vi "se_mot_calc.vi"(6 "targetValid":bool=TRUE, 7 "resetOrigin":bool, 8 "inputValid":bool, 9 "interpOutput":fxp<+/-,19,2>, 10 "origin":T2, 11 "se.mot.p.target":cluster{"x":fxp<+/-,16,1>, "y":fxp<+/-,16,1>}) -> (0 "outputValid":bool, 2 "outputNorm":T1, 3 "outputInt":cluster{"x":i16, "y":i16})   [LabVIEW 2016]
uses:
  <vilib>/rvi/FXPMathLib/FxpSub/XNode/nifxpmath_Sub.xnode
  <vilib>/rvi/FXPMathLib/FxpMul/XNode/nifxpmath_Multiplier.xnode
  <vilib>/rvi/FXPMathLib/FxpAdd/XNode/nifxpmath_Add.xnode
  <vilib>/rvi/FXPMathLib/FxpInterpret/XNode/nifxpmath_Interpret.xnode
  <vilib>/rvi/FXPMathLib/sim/FxpSim.dll
types:
  T1 = cluster{"x+y":fxp<+/-,18,2>, "x+y":fxp<+/-,18,2>}
  T2 = cluster{"xOut":fxp<+/-,18,2>, "yOut":fxp<+/-,18,2>}
  T3 = cluster{"x-y":fxp<+/-,18,2>, "x-y":fxp<+/-,18,2>}
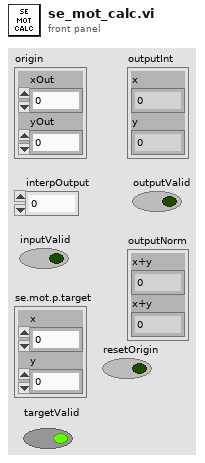
[diagram p1: front panel]
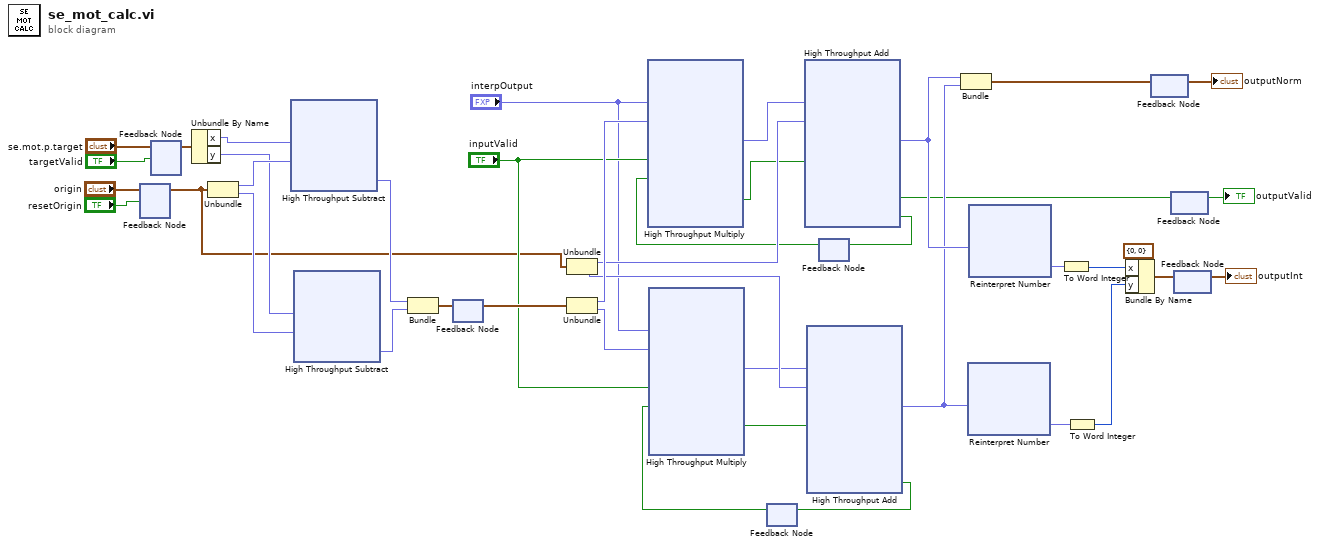
[diagram p0: block diagram]
diagram:
  n1 = feedback-in #1("origin", "resetOrigin") -> ()
  n2 = feedback #1() -> (w2:T2)  [unwired: 1 in]
  n3 = feedback-in #2("se.mot.p.target", "targetValid") -> ()
  n4 = feedback #2() -> (w6:cluster{"x":fxp<+/-,16,1>, "y":fxp<+/-,16,1>})  [unwired: 1 in]
  n5 = Unbundle By Name(w6) -> ("x"=w21:fxp<+/-,16,1>, "y"=w20:fxp<+/-,16,1>)
  n6 = Unbundle(w2) -> ("xOut"=w29:fxp<+/-,18,2>, "yOut"=w28:fxp<+/-,18,2>)
  n7 = xnode "High Throughput Subtract"("x"=w21, "y"=w29) -> ("x-y"=w35:fxp<+/-,18,2>)
  n8 = xnode "High Throughput Subtract"("x"=w20, "y"=w28) -> ("x-y"=w36:fxp<+/-,18,2>)
  n9 = Bundle("x-y"=w35, "x-y"=w36) -> (w37:T3)  [unwired: 1 in]
  n10 = feedback #3() -> (w38:T3)  [unwired: 1 in]
  n11 = feedback-in #3(w37) -> ()
  n12 = Unbundle(w2) -> ("xOut"=w34:fxp<+/-,18,2>, "yOut"=w33:fxp<+/-,18,2>)
  n13 = Unbundle(w38) -> ("x-y"=w41:fxp<+/-,18,2>, "x-y"=w40:fxp<+/-,18,2>)
  n14 = feedback #4() -> (w18:bool)  [unwired: 1 in]
  n15 = xnode ("High Throughput Multiply")("x"="interpOutput", "y"=w40, "input valid"="inputValid", "ready for output (T)"=w18) -> ("x*y"=w13:fxp<+/-,18,2>, "output valid"=w12:bool)  [unwired: 1 out]
  n16 = xnode ("High Throughput Add")("x"=w13, "y"=w33, "input valid"=w12) -> ("x+y"=w25:fxp<+/-,18,2>, "ready for input"=w19:bool)  [unwired: 1 in, 1 out]
  n17 = feedback-in #4(w19) -> ()
  n18 = feedback #5() -> (w16:bool)  [unwired: 1 in]
  n19 = xnode ("High Throughput Multiply")("x"="interpOutput", "y"=w41, "input valid"="inputValid", "ready for output (T)"=w16) -> ("x*y"=w14:fxp<+/-,18,2>, "output valid"=w15:bool)  [unwired: 1 out]
  n20 = xnode ("High Throughput Add")("x"=w14, "y"=w34, "input valid"=w15) -> ("x+y"=w26:fxp<+/-,18,2>, "output valid"=w4:bool, "ready for input"=w17:bool)  [unwired: 1 in]
  n21 = feedback-in #5(w17) -> ()
  n22 = Bundle("x+y"=w26, "x+y"=w25) -> (w27:T1)  [unwired: 1 in]
  n23 = xnode "Reinterpret Number"("x"=w25) -> ("y"=w11:fxp<+/-,18,17>)
  n24 = xnode "Reinterpret Number"("x"=w26) -> ("y"=w8:fxp<+/-,18,17>)
  n25 = To Word Integer(number=w8) -> (16bit integer=w7:i16)
  n26 = To Word Integer(number=w11) -> (16bit integer=w9:i16)
  n27 = Bundle By Name(cluster=cluster{"x":i16, "y":i16} {"x"=0, "y"=0} ("Element"), "x"=w7, "y"=w9) -> (w24:cluster{"x":i16, "y":i16})
  n28 = feedback #6() -> (→"outputNorm":T1)  [unwired: 1 in]
  n29 = feedback-in #6(w27) -> ()
  n30 = feedback #7() -> (→"outputValid":bool)  [unwired: 1 in]
  n31 = feedback-in #7(w4) -> ()
  n32 = feedback #8() -> (→"outputInt":cluster{"x":i16, "y":i16})  [unwired: 1 in]
  n33 = feedback-in #8(w24) -> ()
